vi "Interface_Main.vi"() -> ()   [LabVIEW 2016]
uses:
  Test3(BrRef)_class/Test3(BrRef).lvclass
  Test2(ByValue)_class/Test2(ByValue).lvclass
  Test(ByValue)_class/Test(ByValue).lvclass
  GUID_Interface/GUID.lvclass
  GUID Trait_Interface/GUID Trait.lvclass
  GUID Trait With Attributes_class/GUID Trait With Attributes.lvclass
panel:
  out "error out 4":errorcluster
  out "GUID 3":string
  out "error out 3":errorcluster
  out "GUID 2":string
  out "GUID":string
  out "error out 2":errorcluster
  out "error out":errorcluster
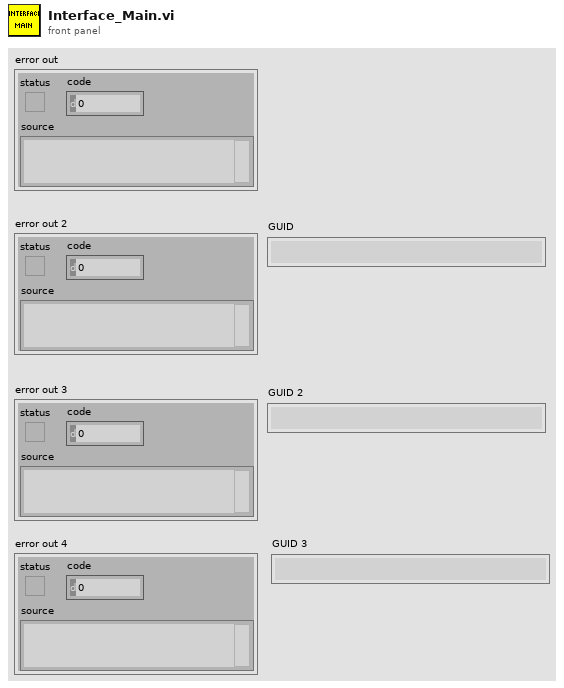
[diagram p1: front panel]
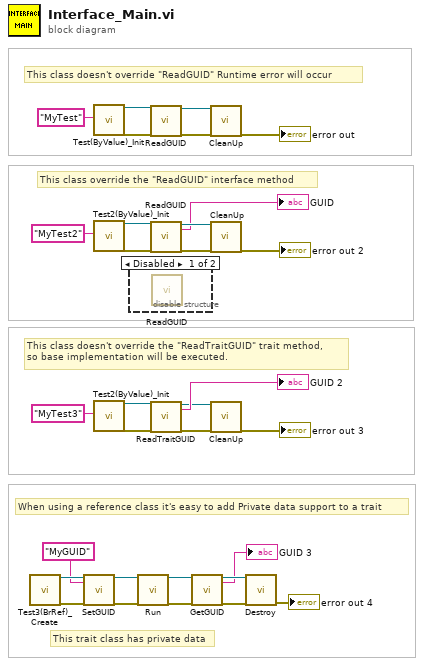
[diagram p0: block diagram]
diagram:
  # "This trait class has private data"
  # "When using a reference class it's easy to add Private data support to a trait"
  # "This class doesn't override the \"ReadTraitGUID\" trait method,\nso base implementation will be executed."
  # "This class override the \"ReadGUID\" interface method"
  # "This class doesn't override \"ReadGUID\" Runtime error will occur"
  n1 = call "Test3(BrRef)_Create.vi"() -> ("reference out"=w11:refnum<class "Test3(BrRef).lvclass">, "error out"=w10:errorcluster)  [unwired: 18 in]
  n2 = call "SetGUID.vi"("Interface In"=w11, "GUID"="MyGUID", "error in (no error)"=w10) -> ("Interface Out"=w9:refnum<class "Test3(BrRef).lvclass">, "error out"=w8:errorcluster)  [unwired: 15 in]
  n3 = call "Test(ByValue)_Init.vi"("TestName"="MyTest") -> ("object out"=w30:refnum<class "Test(ByValue).lvclass">, "error out"=w31:errorcluster)  [unwired: 17 in]
  n4 = call "Test2(ByValue)_Init.vi"("TestName"="MyTest2") -> ("object out"=w21:refnum<class "Test2(ByValue).lvclass">, "error out"=w20:errorcluster)  [unwired: 17 in]
  n5 = call "Test2(ByValue)_Init.vi"("TestName"="MyTest3") -> ("object out"=w16:refnum<class "Test2(ByValue).lvclass">, "error out"=w17:errorcluster)  [unwired: 17 in]
  n6 = disable-structure shown="Disabled" {
    frame Disabled {
      n7 = call-dynamic "ReadGUID.vi"() -> ()  [unwired: 17 in, 3 out]
    }
    frame Enabled {
    }
  }
  n8 = call-dynamic "Run.vi"("reference in"=w9, "error in (no error)"=w8) -> ("reference out"=w6:refnum<class "Test3(BrRef).lvclass">, "error out"=w7:errorcluster)  [unwired: 16 in]
  n9 = call "ReadGUID.vi"("Interface In"=w30, "error in (no error)"=w31) -> ("Interface Out"=w29:refnum<class "Test(ByValue).lvclass">, "error out"=w28:errorcluster)  [unwired: 15 in, 1 out]
  n10 = call "ReadGUID.vi"("Interface In"=w21, "error in (no error)"=w20) -> ("Interface Out"=w22:refnum<class "Test2(ByValue).lvclass">, "GUID"=→"GUID":string, "error out"=w23:errorcluster)  [unwired: 15 in]
  n11 = call "ReadTraitGUID.vi"("Interface In"=w16, "error in (no error)"=w17) -> ("Interface Out"=w15:refnum<class "Test2(ByValue).lvclass">, "GUID"=→"GUID 2":string, "error out"=w14:errorcluster)  [unwired: 15 in]
  n12 = call "GetGUID.vi"("Interface in"=w6, "error in (no error)"=w7) -> ("Interface out"=w5:refnum<class "Test3(BrRef).lvclass">, "GUID"=→"GUID 3":string, "error out"=w4:errorcluster)  [unwired: 15 in]
  n13 = call-dynamic "CleanUp.vi"("object in"=w29, "error in (no error)"=w28) -> ("error out"=→"error out":errorcluster)  [unwired: 16 in, 1 out]
  n14 = call-dynamic "CleanUp.vi"("object in"=w22, "error in (no error)"=w23) -> ("error out"=→"error out 2":errorcluster)  [unwired: 16 in, 1 out]
  n15 = call-dynamic "CleanUp.vi"("object in"=w15, "error in (no error)"=w14) -> ("error out"=→"error out 3":errorcluster)  [unwired: 16 in, 1 out]
  n16 = call-dynamic "Destroy.vi"("reference in"=w5, "error in (no error)"=w4) -> ("error out"=→"error out 4":errorcluster)  [unwired: 16 in, 1 out]
